vi "Write Multiple Registers.vi"(8 "error in (no error)":errorcluster, 9 "values":u16[](array[numeric]), 10 "starting address":u16, 11 "MB session in":refnum<class "MB_Master.lvclass">) -> (0 "error out":errorcluster, 3 "MB session out":refnum<class "MB_Master.lvclass">)   [LabVIEW 2021, in "MB Master.lvlib"]
doc: "Function Code 16: Writes holding register <b>values</b> starting at <b>starting address</b>"
uses:
  <vilib>/Plasmionique/MB Master/MB Master.lvlib
  <vilib>/Plasmionique/MB Master/MB_Master/MB_Master.lvclass
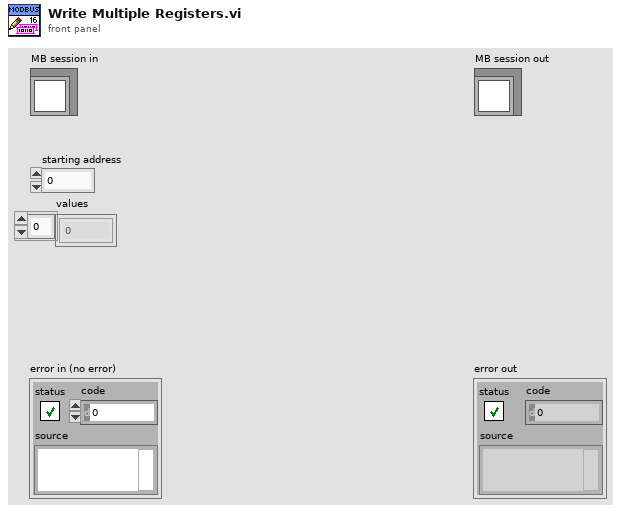
[diagram p1: front panel]
types:
  T1 = typedef "MB Master.lvlib/MB_PDU_Cluster.ctl" = cluster{"Function Code":u8, "Data":u8[], "RTU_DataBytes":i32}
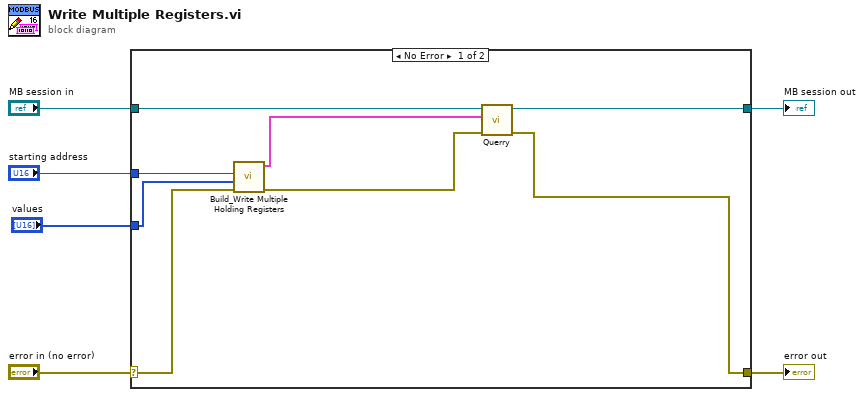
[diagram p0: block diagram]
diagram:
  n1 = case shown="No Error" "error in (no error)" {
    selector: "error in (no error)" -> [w11 w16]
    tunnel: [w10 w16] -> w5
    tunnel: [w13 w15] -> w3
    tunnel: "MB session in" -> [w8 w15]
    tunnel: "starting address" -> [w14 _]
    tunnel: "values" -> [w9 _]
    frame No Error {
      n2 = call <vilib>:"Build_Write Multiple Holding Registers.vi"("error in (no error)"=w11, "values"=w9, "starting address"=w14) -> ("error out"=w12:errorcluster, "MB_PDU"=w7:T1)  [unwired: 7 in]
      n3 = call-dynamic "Querry.vi"("error in (no error)"=w12, "PDU_req"=w7, "MB_Master in"=w8) -> ("error out"=w10:errorcluster, "MB_Master out"=w13:refnum<class "MB_Master.lvclass">)  [unwired: 6 in, 1 out]
    }
    frame Error {
    }
  }
  "error out" <- w5
  "MB session out" <- w3
